vi "Initialise FSM Queue.vi"(8 "error in (no error)":errorcluster) -> (0 "error out":errorcluster)   [LabVIEW 2017]
uses:
  FSM States.ctl
  Application Globals.vi
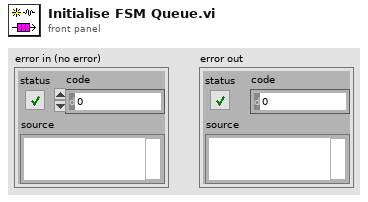
[diagram p1: front panel]
types:
  T1 = typedef "FSM States.ctl" = enum16{"App_Disconnect", "App_Idle", "App_Connect", "App_Close", "APP_Init", "App_Logging", "App_SetRecordStateOn", "App_SetRecordStateOff"}
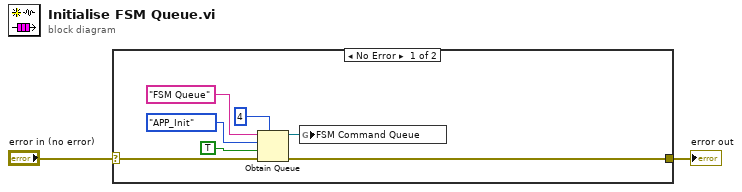
[diagram p0: block diagram]
diagram:
  n1 = case shown="No Error" "error in (no error)" {
    selector: "error in (no error)" -> [w3 w10]
    tunnel: [w9 w10] -> w2
    frame No Error {
      n2 = Obtain Queue(max queue size (-1, unlimited)=4, name (unnamed)="FSM Queue", element data type=FSM_States."APP_Init", create if not found? (T)=TRUE, error in (no error)=w3) -> (queue out=w8:refnum<queue>, error out=w9:errorcluster)  [unwired: 1 out]
      n3 = global write "Application Globals.vi" "FSM Command Queue"(w8) -> ()
    }
    frame Error {
    }
  }
  "error out" <- w2
